vi "thorlabs_disconnect.vi"(8 "error in (no error)":errorcluster, 11 "thorlabs_panel in":refnum<class "thorlabs_panel.lvclass">) -> (0 "error out":errorcluster, 3 "thorlabs_panel out":refnum<class "thorlabs_panel.lvclass">)   [LabVIEW 2015, in "thorlabs_panel.lvclass"]
uses:
  thorlabs_panel.lvclass
  thorlabs_class/thorlabs_kinesis.lvclass
  UI/panel_class/panel.lvclass
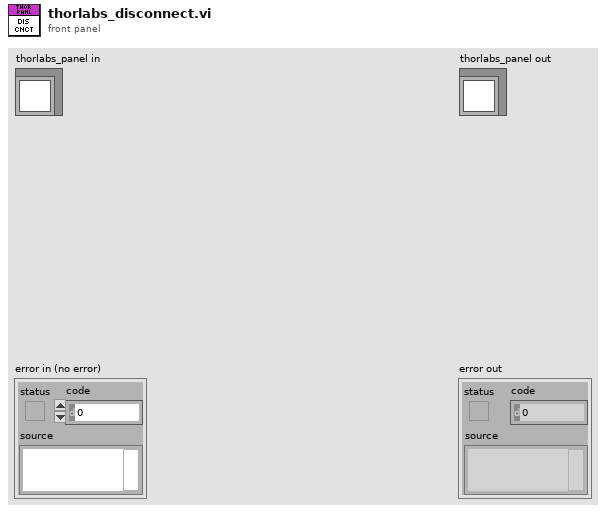
[diagram p1: front panel]
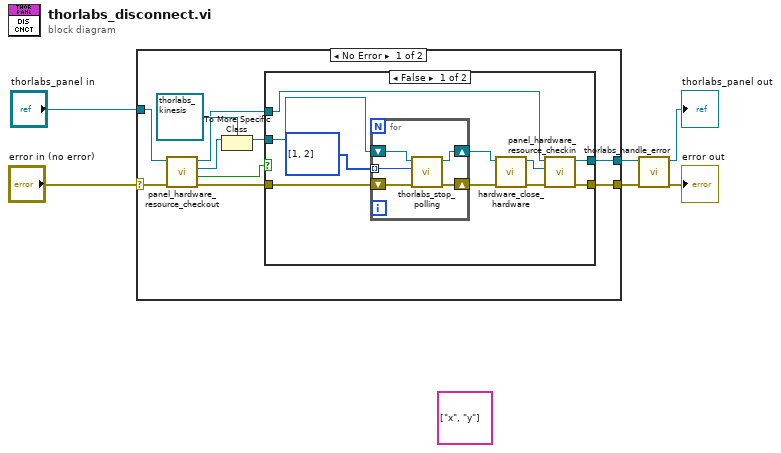
[diagram p0: block diagram]
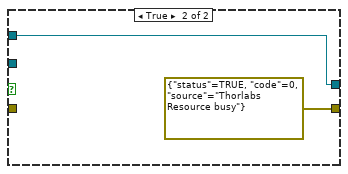
[diagram p2: hidden frame]
diagram:
  (unwired) string[] ["x", "y"]
  n1 = case shown="No Error" "error in (no error)" {
    selector: "error in (no error)" -> [w15 w35]
    tunnel: [w7 w35] -> w3
    tunnel: [w8 w34] -> w4
    tunnel: "thorlabs_panel in" -> [w16 w34]
    frame No Error {
      n2 = call "panel_hardware_resource_checkout.vi"("error in (no error)"=w15, "panel in"=w16) -> ("error out"=w11:errorcluster, "timed out?"=w10:bool, "hardware.lvclass"=w14:refnum<class "hardware.lvclass">, "panel out"=w9:refnum<class "thorlabs_panel.lvclass">)  [unwired: 6 in]
      n3 = To More Specific Class(target class=refnum<class "thorlabs_kinesis.lvclass"> refnum ("thorlabs_kinesis.lvclass"), reference=w14) -> (specific class reference=w12:refnum<class "thorlabs_kinesis.lvclass">)  [unwired: 1 in, 1 out]
      n4 = case shown="False" w10 {
        tunnel: w12 -> [w23 _]
        tunnel: w11 -> [w22 _]
        tunnel: w9 -> [w24 w32]
        tunnel: [w26 w32] -> w8
        tunnel: [w25 errorcluster {"status"=TRUE, "code"=0, "source"="Thorlabs Resource busy"} ("error out")] -> w7
        frame False {
          n5 = for {
            tunnel: i32[] [1, 2] -> [w31] mode=indexing
            shift-right: [w28] -> w21
            shift-left: w22 -> [w29]
            shift-right: [w27] -> w20
            shift-left: w23 -> [w30]
            n6 = call "thorlabs_stop_polling.vi"("error in (no error)"=w29, "channel"=w31, "thorlabs_kinesis in"=w30) -> ("error out"=w28:errorcluster, "thorlabs_kinesis out"=w27:refnum<class "thorlabs_kinesis.lvclass">)  [unwired: 7 in]
          }
          n7 = call-dynamic "hardware_close_hardware.vi"("error in (no error)"=w21, "thorlabs_kinesis in"=w20) -> ("error out"=w18:errorcluster, "thorlabs_kinesis out"=w19:refnum<class "thorlabs_kinesis.lvclass">)  [unwired: 8 in]
          n8 = call "panel_hardware_resource_checkin.vi"("error in (no error)"=w18, "hardware.lvclass"=w19, "panel in"=w24) -> ("error out"=w25:errorcluster, "panel out"=w26:refnum<class "thorlabs_panel.lvclass">)  [unwired: 7 in]
        }
        frame True {
        }
      }
    }
    frame Error {
    }
  }
  n9 = call "thorlabs_handle_error.vi"("error in (no error)"=w3, "thorlabs_panel in"=w4) -> ("error out"=→"error out":errorcluster, "thorlabs_panel out"=→"thorlabs_panel out":refnum<class "thorlabs_panel.lvclass">)  [unwired: 8 in]
